vi "fileObjectivesRegistrationSaveMulti.vi"(1 "z(opto)z(img)":dbl[][](array[numeric]), 2 "z(opto,img) of xy registrations":dbl[][](array[numeric]), 3 "denormParam":dbl[][](array[numeric]), 4 "normParam":dbl[][](array[numeric]), 5 "param":dbl[][][](array[numeric]), 6 "xyz(opto)xyz(img)":dbl[][][](array[numeric])) -> ()   [LabVIEW 2017]
uses:
  globalUtilities.vi
  <vilib>/Utility/file.llb/Write Delimited Spreadsheet (DBL).vi
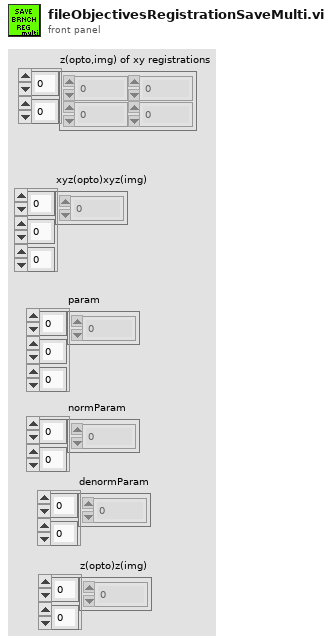
[diagram p1: front panel]
types:
  T1 = enum16{"open", "replace", "create", "open or create", "replace or create", "replace or create with confirmation"}
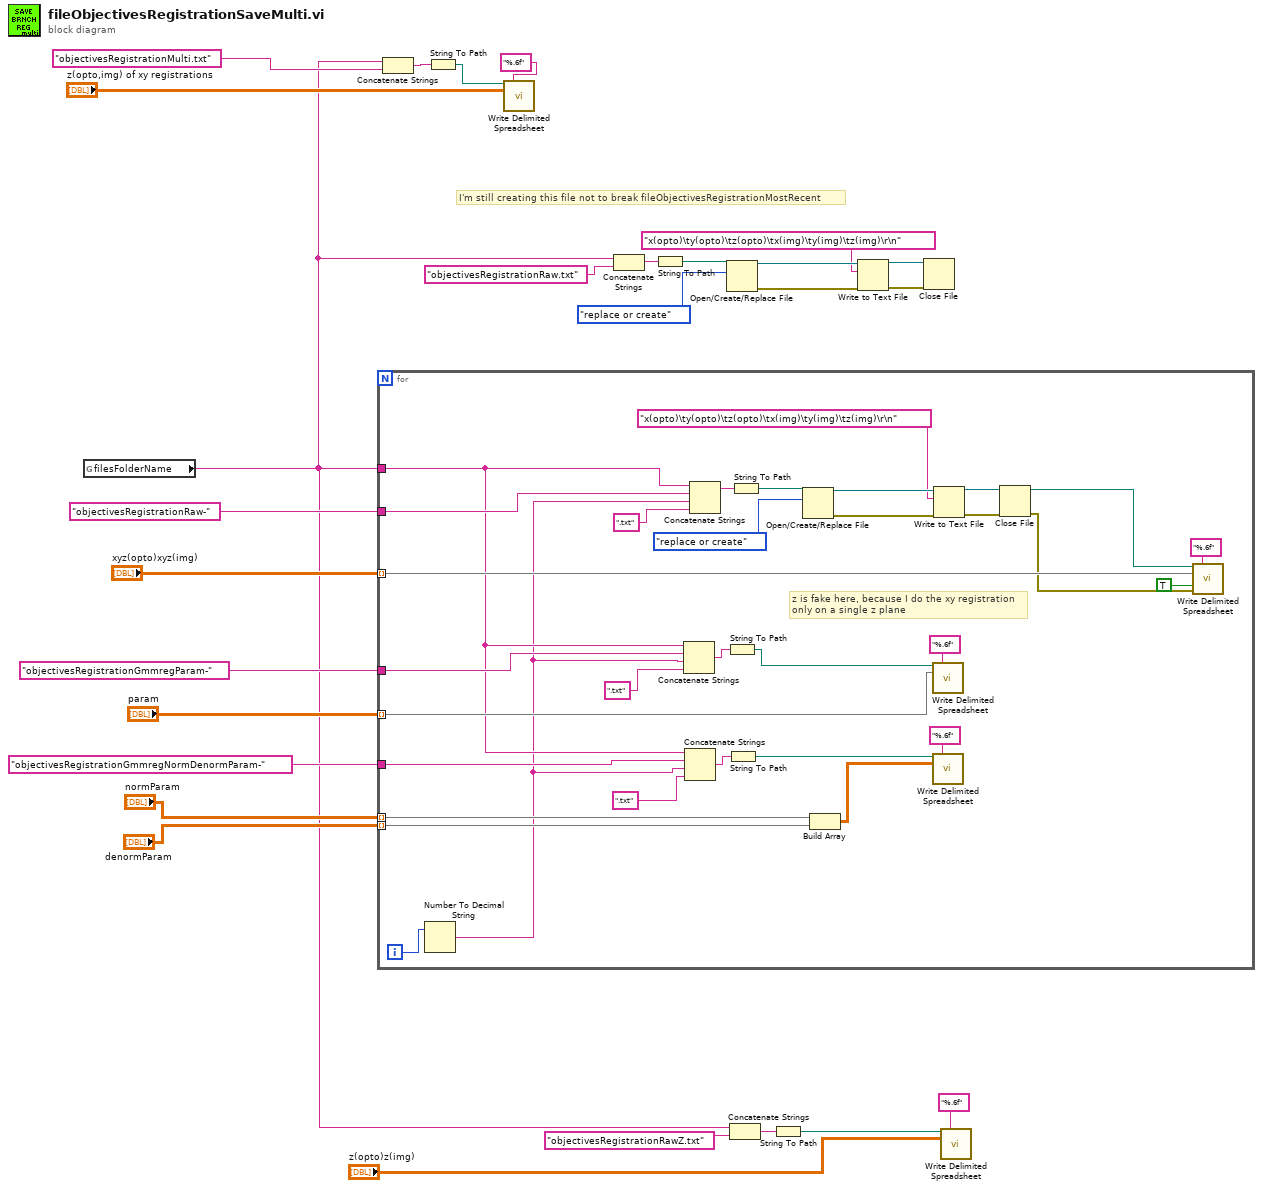
[diagram p0: block diagram]
diagram:
  # "I'm still creating this file not to break fileObjectivesRegistrationMostRecent"
  n1 = global read "globalUtilities.vi" "filesFolderName"() -> (w2:string)
  n2 = for {
    tunnel: "xyz(opto)xyz(img)" -> [w58] mode=indexing
    tunnel: "objectivesRegistrationRaw-" ("string") -> [w50]
    tunnel: "objectivesRegistrationGmmregParam-" ("string") -> [w44]
    tunnel: "param" -> [w41] mode=indexing
    tunnel: "objectivesRegistrationGmmregNormDenormParam-" ("string") -> [w40]
    tunnel: "normParam" -> [w39] mode=indexing
    tunnel: "denormParam" -> [w38] mode=indexing
    tunnel: w2 -> [w33]
    i -> [w31]
    # "z is fake here, because I do the xy registration\nonly on a single z plane"
    n3 = Number To Decimal String(number=w31) -> (decimal integer string=w28:string)  [unwired: 1 in]
    n4 = Concatenate Strings(w33, w44, w28, ".txt") -> (w43:string)
    n5 = Concatenate Strings(w33, w40, w28, ".txt") -> (w36:string)
    n6 = Concatenate Strings(w33, w50, w28, ".txt") -> (w49:string)
    n7 = String To Path(string=w43) -> (path=w42:path)
    n8 = String To Path(string=w36) -> (path=w35:path)
    n9 = String To Path(string=w49) -> (path=w48:path)
    n10 = Open/Create/Replace File(file path (use dialog)=w48, operation (0:open)=T1."replace or create") -> (refnum out=w56:refnum<file>, error out=w53:errorcluster)  [unwired: 4 in, 1 out]
    n11 = Build Array(w39, w38) -> (w34:dbl[][])
    n12 = call-poly <vilib>:"Write Delimited Spreadsheet.vi"("file path (dialog if empty)"=w42, "format (%.3f)"="%.6f", "2D data"=w41) -> ()  [unwired: 11 in, 2 out]
    n13 = call-poly <vilib>:"Write Delimited Spreadsheet.vi"("file path (dialog if empty)"=w35, "format (%.3f)"="%.6f", "2D data"=w34) -> ()  [unwired: 11 in, 2 out]
    n14 = Write to Text File(file (use dialog)=w56, text="x(opto)\ty(opto)\tz(opto)\tx(img)\ty(img)\tz(img)\r\n", error in=w53) -> (refnum out=w54:refnum<file>, error out=w52:errorcluster)  [unwired: 1 in, 1 out]
    n15 = Close File(refnum=w54, error in=w52) -> (path=w46:path, error out=w51:errorcluster)
    n16 = call-poly <vilib>:"Write Delimited Spreadsheet.vi"("file path (dialog if empty)"=w46, "format (%.3f)"="%.6f", "2D data"=w58, "append to file? (new file:F)"=TRUE, "error in (no error)"=w51) -> ()  [unwired: 9 in, 2 out]
  }
  n17 = Concatenate Strings(w2, "objectivesRegistrationMulti.txt" ("string")) -> (w12:string)
  n18 = String To Path(string=w12) -> (path=w11:path)
  n19 = call-poly <vilib>:"Write Delimited Spreadsheet.vi"("file path (dialog if empty)"=w11, "format (%.3f)"="%.6f", "2D data"="z(opto,img) of xy registrations") -> ()  [unwired: 11 in, 2 out]
  n20 = Concatenate Strings(w2, "objectivesRegistrationRaw.txt" ("string")) -> (w5:string)
  n21 = String To Path(string=w5) -> (path=w4:path)
  n22 = Open/Create/Replace File(file path (use dialog)=w4, operation (0:open)=T1."replace or create") -> (refnum out=w10:refnum<file>, error out=w7:errorcluster)  [unwired: 4 in, 1 out]
  n23 = Concatenate Strings(w2, "objectivesRegistrationRawZ.txt" ("string")) -> (w19:string)
  n24 = String To Path(string=w19) -> (path=w17:path)
  n25 = Write to Text File(file (use dialog)=w10, text="x(opto)\ty(opto)\tz(opto)\tx(img)\ty(img)\tz(img)\r\n", error in=w7) -> (refnum out=w8:refnum<file>, error out=w6:errorcluster)  [unwired: 1 in, 1 out]
  n26 = Close File(refnum=w8, error in=w6) -> ()  [unwired: 2 out]
  n27 = call-poly <vilib>:"Write Delimited Spreadsheet.vi"("file path (dialog if empty)"=w17, "format (%.3f)"="%.6f", "2D data"="z(opto)z(img)") -> ()  [unwired: 11 in, 2 out]
